vi "ADD SALE ITEM.vi"(9 "Item Name":string, 10 "Item Price":string, 11 "REFERENCES":T1) -> ()   [LabVIEW 2019]
uses:
  Controls/References Cluster.ctl
  <vilib>/userDefined/High Color/IMAQdx.ctl
  Controls/Custom Calendar/Custom Calendar.xctl
  Controls/Table Data Types/PSC Sales Item Data Type.ctl
  <vilib>/addons/database/Connection.llb/DB Tools Open Connec (String).vi
  <vilib>/addons/database/_DB Variant To Data/Database Variant To Data.xnode
  <vilib>/addons/database/NI_Database_API.lvlib
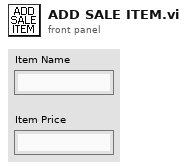
[diagram p1: front panel]
types:
  T1 = typedef "References Cluster.ctl" = cluster{"MAIN PAGES":refnum<vi>, "ADD/EDIT ITEM REFERENCES":cluster{"Identifier":refnum<vi>, "BYU ICN #":refnum<vi>, "Item Description":refnum<vi>, "Comments":refnum<vi>, "Checked Out Date":refnum<vi>, "Due Date":refnum<vi>, "Check Out Location":refnum<vi>, "Reminder Count":refnum<vi>, "Most Recent Reminder Date":refnum<vi>, "BYU ID #":refnum<vi>, "Building/Room":refnum<vi>, "Location in Room":refnum<vi>, "Manual":refnum<vi>, "Manufacturer":refnum<vi>, "Model #":refnum<vi>, "Serial #":refnum<vi>, "Date Acquired":refnum<vi>, "ADD/EDIT ITEM LABEL":refnum<vi>, "ARCHIVE ITEM":refnum<vi>, "Archive Item Inputs":refnum<vi>, "Reminder Notes":refnum<vi>}, "ADD/EDIT USER REFERENCES":cluster{"BYU ID # (##-###-####)":refnum<vi>, "First Name":refnum<vi>, "Last Name":refnum<vi>, "Phone Number (###-###-####)":refnum<vi>, "Email":refnum<vi>, "Department":refnum<vi>, "Graduation Status":refnum<vi>, "Anticipated Graduation Year":refnum<vi>, "Credit Score":refnum<vi>, "Date Added":refnum<vi>, "Graduation Clearance Date":refnum<vi>, "Picture File Name":refnum<vi>, "ADD/EDIT USER LABEL":refnum<vi>, "Department Map":refnum<vi>, "Status Map":refnum<vi>, "Anticipated Graduation Year Map":refnum<vi>, "User Agreement":refnum<vi>, "User Comments":refnum<vi>, "Camera":refnum<vi>}, "RETURN ITEM REFERENCES":cluster{"Item or Person:":refnum<vi>, "Search Return Results":refnum<vi>, "What are you searching for?":refnum<vi>}, "SEARCH DATABASE REFERENCES":cluster{"What to Search For:":refnum<vi>, "Where to Search":refnum<vi>, "Column to Search In":refnum<vi>, "Column to Sort By":refnum<vi>, "Search Database Results":refnum<vi>, "Inventory Column Selector":refnum<vi>, "User Column Selector":refnum<vi>, "Inventory Archive Column Selector":refnum<vi>, "User Archive Column Selector":refnum<vi>, "Sales Tracking Column Selector":refnum<vi>, "Checked In Archive Column Selector":refnum<vi>, "Restore User":refnum<vi>, "Date Range":refnum<vi>, "Dates Less Than":refnum<vi>, "Dates Greater Than":refnum<vi>, "Search Print Receipt":refnum<vi>, "Edit Sale Description":refnum<vi>}, "USER ITEMS REFERENCES":cluster{"USER'S INFORMATION":refnum<vi>, "User's Checked Out Items":refnum<vi>, "User Info Comments":refnum<vi>, "SEE USER INFO COMMENTS":refnum<vi>}, "EDIT ITEMS REFERENCES":cluster{"New Check Out Location":refnum<vi>, "Items to Edit":refnum<vi>, "Edit Items Due Date":refnum<vi>, "New Reminder Notes":refnum<vi>, "New Item Description":refnum<vi>}, "CHECK OUT ITEMS REFERENCES":cluster{"Enter Item:":refnum<vi>, "Check Out Items Due Date":refnum<vi>, "Check Out Location":refnum<vi>, "Items to be Checked Out":refnum<vi>, "Possible Items":refnum<vi>, "Altered Item Description":refnum<vi>}, "TRANSFER ITEMS REFERENCES":cluster{"Search Parameter":refnum<vi>, "What to Match":refnum<vi>, "Matching Individuals":refnum<vi>, "Items to be Transferred":refnum<vi>}, "SETTINGS REFERENCES":cluster{"PSC Database Settings":refnum<vi>, "PSC Sales Item Spreadsheet":refnum<vi>}, "PSC SALES REFERENCES":cluster{"BYU ID CARD #":refnum<vi>, "Sale Description":refnum<vi>, "Scan or Enter Item Name":refnum<vi>, "Items to be Sold":refnum<vi>, "Grand Total":refnum<vi>, "Item List":refnum<vi>}}
  T2 = typedef "PSC Sales Item Data Type.ctl" = cluster{"Item Name":string, "Item Price":string}
  T3 = cluster{"PSC Database Settings":refnum<vi>, "PSC Sales Item Spreadsheet":refnum<vi>}
  T4 = typedef "NI_Database_API.lvlib/Conn ObjectReference.ctl" = refnum<k1>
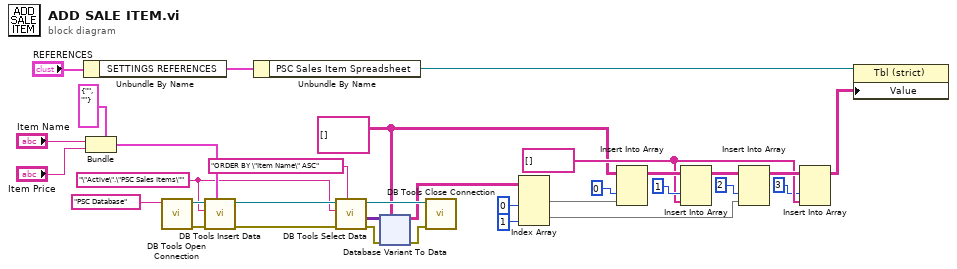
[diagram p0: block diagram]
diagram:
  w6 = string[] []
  w3 = string[][] []
  w18 = "\"Active\".\"PSC Sales Items\"" ("String")
  n1 = Unbundle By Name("REFERENCES") -> ("SETTINGS REFERENCES"=w32:T3)
  n2 = Bundle(cluster=T2 {"Item Name"="", "Item Price"=""}, "Item Name"="Item Name", "Item Price"="Item Price") -> (w25:T2)
  n3 = call-poly <vilib>:"DB Tools Open Connection.vi"("connection information"="PSC Database" ("String")) -> ("error out"=w26:errorcluster, "connection reference"=w27:T4)  [unwired: 7 in]
  n4 = call <vilib>:"DB Tools Insert Data.vi"("data"=w25, "error in (no error)"=w26, "table"=w18, "connection reference"=w27) -> ("error out"=w20:errorcluster, "connection reference out"=w19:T4)  [unwired: 6 in]
  n5 = Unbundle By Name(w32) -> ("PSC Sales Item Spreadsheet"=w2:refnum<vi>)
  n6 = call <vilib>:"DB Tools Select Data.vi"("condition"="ORDER BY \"Item Name\" ASC", "error in (no error)"=w20, "table"=w18, "connection reference"=w19) -> ("error out"=w23:errorcluster, "data"=w24:variant[][], "connection reference out"=w22:T4)  [unwired: 2 in]
  n7 = xnode "Database Variant To Data"("database variant"=w24, "error in (no error)"=w23, "type"=w3) -> ("data"=w4:string[][], "error out"=w21:errorcluster)
  n8 = call <vilib>:"DB Tools Close Connection.vi"("error in (no error)"=w21, "connection reference"=w22) -> ()  [unwired: 5 in, 1 out]
  n9 = Index Array(array=w4, index (col) #1=0 ("disabled index (col)"), index (col) #2=1 ("index (col)")) -> (element #1=w12:string[], element #2=w8:string[])  [unwired: 2 in]
  n10 = Insert Into Array(array=w3, index (col)=0 ("disabled index (col)"), new element=w12) -> (w13:string[][])  [unwired: 1 in]
  n11 = Insert Into Array(array=w13, index (col)=1 ("disabled index (col)"), new element=w6) -> (w10:string[][])  [unwired: 1 in]
  n12 = Insert Into Array(array=w10, index (col)=2 ("disabled index (col)"), new element=w8) -> (w7:string[][])  [unwired: 1 in]
  n13 = Insert Into Array(array=w7, index (col)=3 ("disabled index (col)"), new element=w6) -> (w1:string[][])  [unwired: 1 in]
  n14 = property class="Tbl (strict)"(reference=w2, "Value"=w1) -> ()  [unwired: 1 in, 2 out]
